vi "GeoData.vi"() -> ()   [LabVIEW 2017] (continued)
ND\tStark County\tH1\n58622\t38089\tBelfield\tND\tStark County\tH1\n58641\t38089\tLefor\tND\tStark County\tH1\n58602\t38089\tDickinson\tND\tStark County\tH1\n58652\t38089\tRichardton\tND\tStark County\tH1\n58630\t38089\tGladstone\tND\tStark County\tH1\n58274\t38091\tPortland\tND\tSteele County\tH1\n58035\t38091\tGalesburg\tND\tSteele County\tH1\n58056\t38091\tLuverne\tND\tSteele County\tH1\n58267\t38091\tNorthwood\tND\tSteele County\tH1\n58240\t38091\tHatton\tND\tSteele County\tH1\n58016\t38091\tClifford\tND\tSteele County\tH1\n58277\t38091\tSharon\tND\tSteele County\tH1\n58046\t38091\tHope\tND\tSteele County\tH1\n58230\t38091\tFinley\tND\tSteele County\tH1\n58425\t38091\tCooperstown\tND\tSteele County\tH1\n58401\t38093\tJamestown\tND\tStutsman County\tH1\n58492\t38093\tWimbledon\tND\tStutsman County\tH1\n58472\t38093\tMontpelier\tND\tStutsman County\tH1\n58420\t38093\tBuchanan\tND\tStutsman County\tH1\n58421\t38093\tCarrington\tND\tStutsman County\tH1\n58467\t38093\tMedina\tND\tStutsman County\tH1\n58466\t38093\tMarion\tND\tStutsman County\tH1\n58481\t38093\tSpiritwood\tND\tStutsman County\tH1\n58402\t38093\tJamestown\tND\tStutsman County\tH1\n58476\t38093\tPingree\tND\tStutsman County\tH1\n58483\t38093\tStreeter\tND\tStutsman County\tH1\n58497\t38093\tYpsilanti\tND\tStutsman County\tH1\n58426\t38093\tCourtenay\tND\tStutsman County\tH1\n58475\t38093\tPettibone\tND\tStutsman County\tH1\n58454\t38093\tJud\tND\tStutsman County\tH1\n58405\t38093\tJamestown\tND\tStutsman County\tH1\n58496\t38093\tWoodworth\tND\tStutsman County\tH1\n58424\t38093\tCleveland\tND\tStutsman County\tH1\n58455\t38093\tKensal\tND\tStutsman County\tH1\n58486\t38093\tSykeston\tND\tStutsman County\tH1\n58442\t38093\tGackle\tND\tStutsman County\tH1\n58367\t38095\tRolla\tND\tTowner County\tH1\n58324\t38095\tCando\tND\tTowner County\tH1\n58377\t38095\tStarkweather\tND\tTowner County\tH1\n58339\t38095\tHansboro\tND\tTowner County\tH1\n58352\t38095\tMunich\tND\tTowner County\tH1\n58331\t38095\tEgeland\tND\tTowner County\tH1\n58363\t38095\tPerth\tND\tTowner County\tH1\n58365\t38095\tRocklake\tND\tTowner County\tH1\n58325\t38095\tChurchs ferry\tND\tTowner County\tH1\n58317\t38095\tBisbee\tND\tTowner County\tH1\n58310\t38095\tAgate\tND\tTowner County\tH1\n58346\t38095\tLeeds\tND\tTowner County\tH1\n58372\t38095\tSarles\tND\tTowner County\tH1\n58323\t38095\tCalvin\tND\tTowner County\tH1\n58045\t38097\tHillsboro\tND\tTraill County\tH1\n58274\t38097\tPortland\tND\tTraill County\tH1\n58038\t38097\tGrandin\tND\tTraill County\tH1\n58218\t38097\tBuxton\tND\tTraill County\tH1\n58035\t38097\tGalesburg\tND\tTraill County\tH1\n58009\t38097\tBlanchard\tND\tTraill County\tH1\n58275\t38097\tReynolds\tND\tTraill County\tH1\n58223\t38097\tCummings\tND\tTraill County\tH1\n58240\t38097\tHatton\tND\tTraill County\tH1\n58016\t38097\tClifford\tND\tTraill County\tH1\n58048\t38097\tHunter\tND\tTraill County\tH1\n58257\t38097\tMayville\tND\tTraill County\tH1\n58219\t38097\tCaledonia\tND\tTraill County\tH1\n58259\t38099\tMichigan\tND\tWalsh County\tH1\n58261\t38099\tMinto\tND\tWalsh County\tH1\n58250\t38099\tLankin\tND\tWalsh County\tH1\n58330\t38099\tEdmore\tND\tWalsh County\tH1\n58321\t38099\tBrocket\tND\tWalsh County\tH1\n58227\t38099\tEdinburg\tND\tWalsh County\tH1\n58237\t38099\tGrafton\tND\tWalsh County\tH1\n58231\t38099\tFordville\tND\tWalsh County\tH1\n58224\t38099\tDahlen\tND\tWalsh County\tH1\n58345\t38099\tLawton\tND\tWalsh County\tH1\n58273\t38099\tPisek\tND\tWalsh County\tH1\n58270\t38099\tPark river\tND\tWalsh County\tH1\n58210\t38099\tAdams\tND\tWalsh County\tH1\n58243\t38099\tHoople\tND\tWalsh County\tH1\n58229\t38099\tFairdale\tND\tWalsh County\tH1\n58225\t38099\tDrayton\tND\tWalsh County\tH1\n58233\t38099\tForest river\tND\tWalsh County\tH1\n58779\t38101\tRyder\tND\tWard County\tH1\n58768\t38101\tNorwich\tND\tWard County\tH1\n58731\t38101\tDeering\tND\tWard County\tH1\n58759\t38101\tMax\tND\tWard County\tH1\n58740\t38101\tGlenburn\tND\tWard County\tH1\n58771\t38101\tPlaza\tND\tWard County\tH1\n58756\t38101\tMakoti\tND\tWard County\tH1\n58707\t38101\tMinot\tND\tWard County\tH1\n58704\t38101\tMinot afb\tND\tWard County\tH1\n58718\t38101\tBerthold\tND\tWard County\tH1\n58716\t38101\tBenedict\tND\tWard County\tH1\n58734\t38101\tDonnybrook\tND\tWard County\tH1\n58787\t38101\tTolley\tND\tWard County\tH1\n58721\t38101\tBowbells\tND\tWard County\tH1\n58781\t38101\tSawyer\tND\tWard County\tH1\n58725\t38101\tCarpio\tND\tWard County\tH1\n58733\t38101\tDes lacs\tND\tWard County\tH1\n58703\t38101\tMinot\tND\tWard County\tH1\n58722\t38101\tBurlington\tND\tWard County\tH1\n58790\t38101\tVelva\tND\tWard County\tH1\n58702\t38101\tMinot\tND\tWard County\tH1\n58735\t38101\tDouglas\tND\tWard County\tH1\n58705\t38101\tMinot afb\tND\tWard County\tH1\n58701\t38101\tMinot\tND\tWard County\tH1\n58746\t38101\tKenmare\tND\tWard County\tH1\n58785\t38101\tSurrey\tND\tWard County\tH1\n58374\t38103\tSheyenne\tND\tWells County\tH1\n58348\t38103\tMaddock\tND\tWells County\tH1\n58421\t38103\tCarrington\tND\tWells County\tH1\n58438\t38103\tFessenden\tND\tWells County\tH1\n58422\t38103\tCathay\tND\tWells County\tH1\n58418\t38103\tBowdon\tND\tWells County\tH1\n58356\t38103\tNew rockford\tND\tWells County\tH1\n58423\t38103\tChaseley\tND\tWells County\tH1\n58341\t38103\tHarvey\tND\tWells County\tH1\n58758\t38103\tMartin\tND\tWells County\tH1\n58486\t38103\tSykeston\tND\tWells County\tH1\n58451\t38103\tHurdsfield\tND\tWells County\tH1\n58801\t38105\tWilliston\tND\tWilliams County\tH1\n58849\t38105\tRay\tND\tWilliams County\tH1\n58845\t38105\tGrenora\tND\tWilliams County\tH1\n58843\t38105\tEpping\tND\tWilliams County\tH1\n58802\t38105\tWilliston\tND\tWilliams County\tH1\n58856\t38105\tZahl\tND\tWilliams County\tH1\n58755\t38105\tMcgregor\tND\tWilliams County\tH1\n58830\t38105\tAlamo\tND\tWilliams County\tH1\n58795\t38105\tWildrose\tND\tWilliams County\tH1\n58803\t38105\tWilliston\tND\tWilliams County\tH1\n58853\t38105\tTrenton\tND\tWilliams County\tH1\n58794\t38105\tWhite earth\tND\tWilliams County\tH1\n58852\t38105\tTioga\tND\tWilliams County\tH1\n45660\t39001\tPeebles\tOH\tAdams County\tH1\n45693\t39001\tWest union\tOH\tAdams County\tH1\n45144\t39001\tManchester\tOH\tAdams County\tH1\n45618\t39001\tCherry fork\tOH\tAdams County\tH1\n45616\t39001\tBlue creek\tOH\tAdams County\tH1\n45697\t39001\tWinchester\tOH\tAdams County\tH1\n45684\t39001\tStout\tOH\tAdams County\tH1\n45650\t39001\tLynx\tOH\tAdams County\tH1\n45101\t39001\tAberdeen\tOH\tAdams County\tH1\n45679\t39001\tSeaman\tOH\tAdams County\tH1\n45671\t39001\tRarden\tOH\tAdams County\tH1\n45105\t39001\tBentonville\tOH\tAdams County\tH1\n45657\t39001\tOtway\tOH\tAdams County\tH1\n45801\t39003\tLima\tOH\tAllen County\tH1\n45810\t39003\tAda\tOH\tAllen County\tH1\n45830\t39003\tColumbus grove\tOH\tAllen County\tH1\n45806\t39003\tLima\tOH\tAllen County\tH1\n45807\t39003\tLima\tOH\tAllen County\tH1\n45850\t39003\tHarrod\tOH\tAllen County\tH1\n45877\t39003\tPandora\tOH\tAllen County\tH1\n43310\t39003\tBelle center\tOH\tAllen County\tH1\n45802\t39003\tLima\tOH\tAllen County\tH1\n45854\t39003\tLafayette\tOH\tAllen County\tH1\n45895\t39003\tWapakoneta\tOH\tAllen County\tH1\n45896\t39003\tWaynesfield\tOH\tAllen County\tH1\n45833\t39003\tDelphos\tOH\tAllen County\tH1\n45805\t39003\tLima\tOH\tAllen County\tH1\n45881\t39003\tRawson\tOH\tAllen County\tH1\n45844\t39003\tFort jennings\tOH\tAllen County\tH1\n45820\t39003\tCairo\tOH\tAllen County\tH1\n45817\t39003\tBluffton\tOH\tAllen County\tH1\n45808\t39003\tBeaverdam\tOH\tAllen County\tH1\n45894\t39003\tVenedocia\tOH\tAllen County\tH1\n45887\t39003\tSpencerville\tOH\tAllen County\tH1\n45809\t39003\tGomer\tOH\tAllen County\tH1\n45804\t39003\tLima\tOH\tAllen County\tH1\n45812\t39003\tAlger\tOH\tAllen County\tH1\n44843\t39005\tLucas\tOH\tAshland County\tH1\n44864\t39005\tPerrysville\tOH\tAshland County\tH1\n44859\t39005\tNova\tOH\tAshland County\tH1\n44866\t39005\tPolk\tOH\tAshland County\tH1\n44287\t39005\tWest salem\tOH\tAshland County\tH1\n44691\t39005\tWooster\tOH\tAshland County\tH1\n44805\t39005\tAshland\tOH\tAshland County\tH1\n44837\t39005\tGreenwich\tOH\tAshland County\tH1\n44235\t39005\tHomerville\tOH\tAshland County\tH1\n44822\t39005\tButler\tOH\tAshland County\tH1\n44838\t39005\tHayesville\tOH\tAshland County\tH1\n44874\t39005\tSavannah\tOH\tAshland County\tH1\n44903\t39005\tMansfield\tOH\tAshland County\tH1\n44878\t39005\tShiloh\tOH\tAshland County\tH1\n44851\t39005\tNew london\tOH\tAshland County\tH1\n44842\t39005\tLoudonville\tOH\tAshland County\tH1\n44880\t39005\tSullivan\tOH\tAshland County\tH1\n44840\t39005\tJeromesville\tOH\tAshland County\tH1\n44848\t39005\tNankin\tOH\tAshland County\tH1\n44638\t39005\tLakeville\tOH\tAshland County\tH1\n44048\t39007\tKingsville\tOH\tAshtabula County\tH1\n44041\t39007\tGeneva\tOH\tAshtabula County\tH1\n44047\t39007\tJefferson\tOH\tAshtabula County\tH1\n44085\t39007\tRome\tOH\tAshtabula County\tH1\n44082\t39007\tPierpont\tOH\tAshtabula County\tH1\n44086\t39007\tThompson\tOH\tAshtabula County\tH1\n44046\t39007\tHuntsburg\tOH\tAshtabula County\tH1\n44084\t39007\tRock creek\tOH\tAshtabula County\tH1\n44032\t39007\tDorset\tOH\tAshtabula County\tH1\n44004\t39007\tAshtabula\tOH\tAshtabula County\tH1\n44003\t39007\tAndover\tOH\tAshtabula County\tH1\n44068\t39007\tNorth kingsville\tOH\tAshtabula County\tH1\n44062\t39007\tMiddlefield\tOH\tAshtabula County\tH1\n44428\t39007\tKinsman\tOH\tAshtabula County\tH1\n44076\t39007\tOrwell\tOH\tAshtabula County\tH1\n44010\t39007\tAustinburg\tOH\tAshtabula County\tH1\n44057\t39007\tMadison\tOH\tAshtabula County\tH1\n44093\t39007\tWilliamsfield\tOH\tAshtabula County\tH1\n44030\t39007\tConneaut\tOH\tAshtabula County\tH1\n44099\t39007\tWindsor\tOH\tAshtabula County\tH1\n44064\t39007\tMontville\tOH\tAshtabula County\tH1\n44088\t39007\tUnionville\tOH\tAshtabula County\tH1\n45701\t39009\tAthens\tOH\tAthens County\tH1\n45778\t39009\tStewart\tOH\tAthens County\tH1\n45780\t39009\tThe plains\tOH\tAthens County\tH1\n45723\t39009\tCoolville\tOH\tAthens County\tH1\n45766\t39009\tNew marshfield\tOH\tAthens County\tH1\n45782\t39009\tTrimble\tOH\tAthens County\tH1\n45776\t39009\tShade\tOH\tAthens County\tH1\n45711\t39009\tAmesville\tOH\tAthens County\tH1\n45732\t39009\tGlouster\tOH\tAthens County\tH1\n45764\t39009\tNelsonville\tOH\tAthens County\tH1\n45735\t39009\tGuysville\tOH\tAthens County\tH1\n45739\t39009\tHockingport\tOH\tAthens County\tH1\n43728\t39009\tChesterhill\tOH\tAthens County\tH1\n45710\t39009\tAlbany\tOH\tAthens County\tH1\n45742\t39009\tLittle hocking\tOH\tAthens County\tH1\n45761\t39009\tMillfield\tOH\tAthens County\tH1\n45716\t39009\tBuchtel\tOH\tAthens County\tH1\n45740\t39009\tJacksonville\tOH\tAthens County\tH1\n45719\t39009\tChauncey\tOH\tAthens County\tH1\n45801\t39011\tLima\tOH\tAuglaize County\tH1\n45865\t39011\tMinster\tOH\tAuglaize County\tH1\n43331\t39011\tLakeview\tOH\tAuglaize County\tH1\n45862\t39011\tMendon\tOH\tAuglaize County\tH1\n45806\t39011\tLima\tOH\tAuglaize County\tH1\n45850\t39011\tHarrod\tOH\tAuglaize County\tH1\n45888\t39011\tUniopolis\tOH\tAuglaize County\tH1\n45306\t39011\tBotkins\tOH\tAuglaize County\tH1\n45854\t39011\tLafayette\tOH\tAuglaize County\tH1\n45822\t39011\tCelina\tOH\tAuglaize County\tH1\n45895\t39011\tWapakoneta\tOH\tAuglaize County\tH1\n45896\t39011\tWaynesfield\tOH\tAuglaize County\tH1\n45871\t39011\tNew knoxville\tOH\tAuglaize County\tH1\n45869\t39011\tNew bremen\tOH\tAuglaize County\tH1\n45819\t39011\tBuckland\tOH\tAuglaize County\tH1\n45885\t39011\tSaint marys\tOH\tAuglaize County\tH1\n45887\t39011\tSpencerville\tOH\tAuglaize County\tH1\n45334\t39011\tJackson center\tOH\tAuglaize County\tH1\n45884\t39011\tSaint johns\tOH\tAuglaize County\tH1\n45845\t39011\tFort loramie\tOH\tAuglaize County\tH1\n45870\t39011\tNew hampshire\tOH\tAuglaize County\tH1\n43906\t39013\tBellaire\tOH\tBelmont County\tH1\n43917\t39013\tDillonvale\tOH\tBelmont County\tH1\n43977\t39013\tFlushing\tOH\tBelmont County\tH1\n43902\t39013\tAlledonia\tOH\tBelmont County\tH1\n43942\t39013\tPowhatan point\tOH\tBelmont County\tH1\n43719\t39013\tBethesda\tOH\tBelmont County\tH1\n43940\t39013\tNeffs\tOH\tBelmont County\tH1\n43943\t39013\tRayland\tOH\tBelmont County\tH1\n43935\t39013\tMartins ferry\tOH\tBelmont County\tH1\n43716\t39013\tBeallsville\tOH\tBelmont County\tH1\n43983\t39013\tPiedmont\tOH\tBelmont County\tH1\n43773\t39013\tQuaker city\tOH\tBelmont County\tH1\n43747\t39013\tJerusalem\tOH\tBelmont County\tH1\n43912\t39013\tBridgeport\tOH\tBelmont County\tH1\n43901\t39013\tAdena\tOH\tBelmont County\tH1\n43973\t39013\tFreeport\tOH\tBelmont County\tH1\n43933\t39013\tJacobsburg\tOH\tBelmont County\tH1\n43985\t39013\tHolloway\tOH\tBelmont County\tH1\n43927\t39013\tFairpoint\tOH\tBelmont County\tH1\n43916\t39013\tColerain\tOH\tBelmont County\tH1\n43905\t39013\tBarton\tOH\tBelmont County\tH1\n43972\t39013\tBannock\tOH\tBelmont County\tH1\n43934\t39013\tLansing\tOH\tBelmont County\tH1\n43971\t39013\tYorkville\tOH\tBelmont County\tH1\n43947\t39013\tShadyside\tOH\tBelmont County\tH1\n43718\t39013\tBelmont\tOH\tBelmont County\tH1\n43951\t39013\tLafferty\tOH\tBelmont County\tH1\n43937\t39013\tMaynard\tOH\tBelmont County\tH1\n43909\t39013\tBlaine\tOH\tBelmont County\tH1\n43950\t39013\tSaint clairsville\tOH\tBelmont County\tH1\n43713\t39013\tBarnesville\tOH\tBelmont County\tH1\n43967\t39013\tWarnock\tOH\tBelmont County\tH1\n43759\t39013\tMorristown\tOH\tBelmont County\tH1\n43928\t39013\tGlencoe\tOH\tBelmont County\tH1\n45119\t39015\tFeesburg\tOH\tBrown County\tH1\n45144\t39015\tManchester\tOH\tBrown County\tH1\n45167\t39015\tRipley\tOH\tBrown County\tH1\n45118\t39015\tFayetteville\tOH\tBrown County\tH1\n45142\t39015\tLynchburg\tOH\tBrown County\tH1\n45148\t39015\tMidland\tOH\tBrown County\tH1\n45121\t39015\tGeorgetown\tOH\tBrown County\tH1\n45697\t39015\tWinchester\tOH\tBrown County\tH1\n45154\t39015\tMount orab\tOH\tBrown County\tH1\n45107\t39015\tBlanchester\tOH\tBrown County\tH1\n45130\t39015\tHamersville\tOH\tBrown County\tH1\n45131\t39015\tHigginsport\tOH\tBrown County\tH1\n45171\t39015\tSardinia\tOH\tBrown County\tH1\n45106\t39015\tBethel\tOH\tBrown County\tH1\n45101\t39015\tAberdeen\tOH\tBrown County\tH1\n45115\t39015\tDecatur\tOH\tBrown County\tH1\n45176\t39015\tWilliamsburg\tOH\tBrown County\tH1\n45133\t39015\tHillsboro\tOH\tBrown County\tH1\n45120\t39015\tFelicity\tOH\tBrown County\tH1\n45168\t39015\tRussellville\tOH\tBrown County\tH1\n45005\t39017\tFranklin\tOH\tButler County\tH1\n45013\t39017\tHamilton\tOH\tButler County\tH1\n45014\t39017\tFairfield\tOH\tButler County\tH1\n45249\t39017\tCincinnati\tOH\tButler County\tH1\n45018\t39017\tFairfield\tOH\tButler County\tH1\n45003\t39017\tCollege corner\tOH\tButler County\tH1\n45069\t39017\tWest chester\tOH\tButler County\tH1\n45067\t39017\tTrenton\tOH\tButler County\tH1\n45071\t39017\tWest chester\tOH\tButler County\tH1\n45053\t39017\tOkeana\tOH\tButler County\tH1\n45030\t39017\tHarrison\tOH\tButler County\tH1\n45327\t39017\tGermantown\tOH\tButler County\tH1\n45063\t39017\tShandon\tOH\tButler County\tH1\n45004\t39017\tCollinsville\tOH\tButler County\tH1\n45064\t39017\tSomerville\tOH\tButler County\tH1\n45062\t39017\tSeven mile\tOH\tButler County\tH1\n45055\t39017\tOverpeck\tOH\tButler County\tH1\n45015\t39017\tHamilton\tOH\tButler County\tH1\n45042\t39017\tMiddletown\tOH\tButler County\tH1\n45044\t39017\tMiddletown\tOH\tButler County\tH1\n45050\t39017\tMonroe\tOH\tButler County\tH1\n45246\t39017\tCincinnati\tOH\tButler County\tH1\n45061\t39017\tRoss\tOH\tButler County\tH1\n45011\t39017\tHamilton\tOH\tButler County\tH1\n45056\t39017\tOxford\tOH\tButler County\tH1\n45241\t39017\tCincinnati\tOH\tButler County\tH1\n45012\t39017\tHamilton\tOH\tButler County\tH1\n44657\t39019\tMinerva\tOH\tCarroll County\tH1\n44695\t39019\tBowerston\tOH\tCarroll County\tH1\n44620\t39019\tDellroy\tOH\tCarroll County\tH1\n44644\t39019\tMalvern\tOH\tCarroll County\tH1\n44607\t39019\tAugusta\tOH\tCarroll County\tH1\n43988\t39019\tScio\tOH\tCarroll County\tH1\n44656\t39019\tMineral city\tOH\tCarroll County\tH1\n44643\t39019\tMagnolia\tOH\tCarroll County\tH1\n43908\t39019\tBergholz\tOH\tCarroll County\tH1\n44621\t39019\tDennison\tOH\tCarroll County\tH1\n44615\t39019\tCarrollton\tOH\tCarroll County\tH1\n43945\t39019\tSalineville\tOH\tCarroll County\tH1\n44651\t39019\tMechanicstown\tOH\tCarroll County\tH1\n44688\t39019\tWaynesburg\tOH\tCarroll County\tH1\n44625\t39019\tEast rochester\tOH\tCarroll County\tH1\n44639\t39019\tLeesville\tOH\tCarroll County\tH1\n43903\t39019\tAmsterdam\tOH\tCarroll County\tH1\n43986\t39019\tJewett\tOH\tCarroll County\tH1\n44730\t39019\tEast canton\tOH\tCarroll County\tH1\n44675\t39019\tSherrodsville\tOH\tCarroll County\tH1\n44427\t39019\tKensington\tOH\tCarroll County\tH1\n43047\t39021\tMingo\tOH\tChampaign County\tH1\n45502\t39021\tSpringfield\tOH\tChampaign County\tH1\n43070\t39021\tRosewood\tOH\tChampaign County\tH1\n43357\t39021\tWest liberty\tOH\tChampaign County\tH1\n45317\t39021\tConover\tOH\tChampaign County\tH1\n43060\t39021\tNorth lewisburg\tOH\tChampaign County\tH1\n43009\t39021\tCable\tOH\tChampaign County\tH1\n43045\t39021\tMilford center\tOH\tChampaign County\tH1\n43083\t39021\tWestville\tOH\tChampaign County\tH1\n45389\t39021\tChristiansburg\tOH\tChampaign County\tH1\n43078\t39021\tUrbana\tOH\tChampaign County\tH1\n43072\t39021\tSaint paris\tOH\tChampaign County\tH1\n43343\t39021\tQuincy\tOH\tChampaign County\tH1\n43318\t39021\tDe graff\tOH\tChampaign County\tH1\n45344\t39021\tNew carlisle\tOH\tChampaign County\tH1\n45365\t39021\tSidney\tOH\tChampaign County\tH1\n43044\t39021\tMechanicsburg\tOH\tChampaign County\tH1\n45312\t39021\tCasstown\tOH\tChampaign County\tH1\n43084\t39021\tWoodstock\tOH\tChampaign County\tH1\n45501\t39023\tSpringfield\tOH\tClark County\tH1\n45369\t39023\tSouth vienna\tOH\tClark County\tH1\n45387\t39023\tYellow springs\tOH\tClark County\tH1\n45502\t39023\tSpringfield\tOH\tClark County\tH1\n45319\t39023\tDonnelsville\tOH\tClark County\tH1\n43140\t39023\tLondon\tOH\tClark County\tH1\n45504\t39023\tSpringfield\tOH\tClark County\tH1\n43153\t39023\tSouth solon\tOH\tClark County\tH1\n45372\t39023\tTremont city\tOH\tClark County\tH1\n43078\t39023\tUrbana\tOH\tClark County\tH1\n45368\t39023\tSouth charleston\tOH\tClark County\tH1\n45349\t39023\tNorth hampton\tOH\tClark County\tH1\n45344\t39023\tNew carlisle\tOH\tClark County\tH1\n45314\t39023\tCedarville\tOH\tClark County\tH1\n45323\t39023\tEnon\tOH\tClark County\tH1\n45503\t39023\tSpringfield\tOH\tClark County\tH1\n45506\t39023\tSpringfield\tOH\tClark County\tH1\n43010\t39023\tCatawba\tOH\tClark County\tH1\n43044\t39023\tMechanicsburg\tOH\tClark County\tH1\n45324\t39023\tFairborn\tOH\tClark County\tH1\n45312\t39023\tCasstown\tOH\tClark County\tH1\n45341\t39023\tMedway\tOH\tClark County\tH1\n45505\t39023\tSpringfield\tOH\tClark County\tH1\n45153\t39025\tMoscow\tOH\tClermont County\tH1\n45255\t39025\tCincinnati\tOH\tClermont County\tH1\n45147\t39025\tMiamiville\tOH\tClermont County\tH1\n45103\t39025\tBatavia\tOH\tClermont County\tH1\n45150\t39025\tMilford\tOH\tClermont County\tH1\n45118\t39025\tFayetteville\tOH\tClermont County\tH1\n45162\t39025\tPleasant plain\tOH\tClermont County\tH1\n45121\t39025\tGeorgetown\tOH\tClermont County\tH1\n45156\t39025\tNeville\tOH\tClermont County\tH1\n45112\t39025\tChilo\tOH\tClermont County\tH1\n45107\t39025\tBlanchester\tOH\tClermont County\tH1\n45130\t39025\tHamersville\tOH\tClermont County\tH1\n45102\t39025\tAmelia\tOH\tClermont County\tH1\n45122\t39025\tGoshen\tOH\tClermont County\tH1\n45157\t39025\tNew richmond\tOH\tClermont County\tH1\n45106\t39025\tBethel\tOH\tClermont County\tH1\n45244\t39025\tCincinnati\tOH\tClermont County\tH1\n45176\t39025\tWilliamsburg\tOH\tClermont County\tH1\n45120\t39025\tFelicity\tOH\tClermont County\tH1\n45245\t39025\tCincinnati\tOH\tClermont County\tH1\n45140\t39025\tLoveland\tOH\tClermont County\tH1\n45160\t39025\tOwensville\tOH\tClermont County\tH1\n45158\t39025\tNewtonsville\tOH\tClermont County\tH1\n45177\t39027\tWilmington\tOH\tClinton County\tH1\n45164\t39027\tPort william\tOH\tClinton County\tH1\n45142\t39027\tLynchburg\tOH\tClinton County\tH1\n45148\t39027\tMidland\tOH\tClinton County\tH1\n45159\t39027\tNew vienna\tOH\tClinton County\tH1\n45169\t39027\tSabina\tOH\tClinton County\tH1\n45385\t39027\tXenia\tOH\tClinton County\tH1\n45146\t39027\tMartinsville\tOH\tClinton County\tH1\n45107\t39027\tBlanchester\tOH\tClinton County\tH1\n45068\t39027\tWaynesville\tOH\tClinton County\tH1\n45113\t39027\tClarksville\tOH\tClinton County\tH1\n45135\t39027\tLeesburg\tOH\tClinton County\tH1\n45335\t39027\tJamestown\tOH\tClinton County\tH1\n45114\t39027\tCuba\tOH\tClinton County\tH1\n43160\t39027\tWashington court house\tOH\tClinton County\tH1\n45166\t39027\tReesville\tOH\tClinton County\tH1\n44657\t39029\tMinerva\tOH\tColumbiana County\tH1\n44455\t39029\tRogers\tOH\tColumbiana County\tH1\n44493\t39029\tWinona\tOH\tColumbiana County\tH1\n44454\t39029\tPetersburg\tOH\tColumbiana County\tH1\n44415\t39029\tElkton\tOH\tColumbiana County\tH1\n44460\t39029\tSalem\tOH\tColumbiana County\tH1\n44408\t39029\tColumbiana\tOH\tColumbiana County\tH1\n44413\t39029\tEast palestine\tOH\tColumbiana County\tH1\n43930\t39029\tHammondsville\tOH\tColumbiana County\tH1\n43962\t39029\tSummitville\tOH\tColumbiana County\tH1\n43945\t39029\tSalineville\tOH\tColumbiana County\tH1\n44634\t39029\tHomeworth\tOH\tColumbiana County\tH1\n44625\t39029\tEast rochester\tOH\tColumbiana County\tH1\n43932\t39029\tIrondale\tOH\tColumbiana County\tH1\n44431\t39029\tLeetonia\tOH\tColumbiana County\tH1\n44445\t39029\tNew waterford\tOH\tColumbiana County\tH1\n44490\t39029\tWashingtonville\tOH\tColumbiana County\tH1\n44443\t39029\tNew springfield\tOH\tColumbiana County\tH1\n43968\t39029\tWellsville\tOH\tColumbiana County\tH1\n44601\t39029\tAlliance\tOH\tColumbiana County\tH1\n44427\t39029\tKensington\tOH\tColumbiana County\tH1\n43920\t39029\tEast liverpool\tOH\tColumbiana County\tH1\n44432\t39029\tLisbon\tOH\tColumbiana County\tH1\n44423\t39029\tHanoverton\tOH\tColumbiana County\tH1\n44441\t39029\tNegley\tOH\tColumbiana County\tH1\n44492\t39029\tWest point\tOH\tColumbiana County\tH1\n44609\t39029\tBeloit\tOH\tColumbiana County\tH1\n44665\t39029\tNorth georgetown\tOH\tColumbiana County\tH1\n43845\t39031\tWest lafayette\tOH\tCoshocton County\tH1\n43828\t39031\tKeene\tOH\tCoshocton County\tH1\n43824\t39031\tFresno\tOH\tCoshocton County\tH1\n43821\t39031\tDresden\tOH\tCoshocton County\tH1\n43749\t39031\tKimbolton\tOH\tCoshocton County\tH1\n44637\t39031\tKillbuck\tOH\tCoshocton County\tH1\n43811\t39031\tConesville\tOH\tCoshocton County\tH1\n43803\t39031\tBakersville\tOH\tCoshocton County\tH1\n44654\t39031\tMillersburg\tOH\tCoshocton County\tH1\n43804\t39031\tBaltic\tOH\tCoshocton County\tH1\n43812\t39031\tCoshocton\tOH\tCoshocton County\tH1\n43832\t39031\tNewcomerstown\tOH\tCoshocton County\tH1\n43844\t39031\tWarsaw\tOH\tCoshocton County\tH1\n43822\t39031\tFrazeysburg\tOH\tCoshocton County\tH1\n43006\t39031\tBrinkhaven\tOH\tCoshocton County\tH1\n43805\t39031\tBlissfield\tOH\tCoshocton County\tH1\n43840\t39031\tStone creek\tOH\tCoshocton County\tH1\n43843\t39031\tWalhonding\tOH\tCoshocton County\tH1\n43836\t39031\tPlainfield\tOH\tCoshocton County\tH1\n44827\t39033\tCrestline\tOH\tCrawford County\tH1\n44887\t39033\tTiro\tOH\tCrawford County\tH1\n44849\t39033\tNevada\tOH\tCrawford County\tH1\n44875\t39033\tShelby\tOH\tCrawford County\tH1\n44860\t39033\tOceola\tOH\tCrawford County\tH1\n43314\t39033\tCaledonia\tOH\tCrawford County\tH1\n44818\t39033\tBloomville\tOH\tCrawford County\tH1\n43302\t39033\tMarion\tOH\tCrawford County\tH1\n44881\t39033\tSulphur springs\tOH\tCrawford County\tH1\n44865\t39033\tPlymouth\tOH\tCrawford County\tH1\n44825\t39033\tChatfield\tOH\tCrawford County\tH1\n44833\t39033\tGalion\tOH\tCrawford County\tH1\n44854\t39033\tNew washington\tOH\tCrawford County\tH1\n44882\t39033\tSycamore\tOH\tCrawford County\tH1\n44856\t39033\tNorth robinson\tOH\tCrawford County\tH1\n44820\t39033\tBucyrus\tOH\tCrawford County\tH1\n44026\t39035\tChesterland\tOH\tCuyahoga County\tH1\n44130\t39035\tCleveland\tOH\tCuyahoga County\tH1\n44111\t39035\tCleveland\tOH\tCuyahoga County\tH1\n44113\t39035\tCleveland\tOH\tCuyahoga County\tH1\n44144\t39035\tCleveland\tOH\tCuyahoga County\tH1\n44102\t39035\tCleveland\tOH\tCuyahoga County\tH1\n44040\t39035\tGates mills\tOH\tCuyahoga County\tH1\n44017\t39035\tBerea\tOH\tCuyahoga County\tH1\n44124\t39035\tCleveland\tOH\tCuyahoga County\tH1\n44109\t39035\tCleveland\tOH\tCuyahoga County\tH1\n44127\t39035\tCleveland\tOH\tCuyahoga County\tH1\n44112\t39035\tCleveland\tOH\tCuyahoga County\tH1\n44136\t39035\tStrongsville\tOH\tCuyahoga County\tH1\n44138\t39035\tOlmsted falls\tOH\tCuyahoga County\tH1\n44143\t39035\tCleveland\tOH\tCuyahoga County\tH1\n44105\t39035\tCleveland\tOH\tCuyahoga County\tH1\n44023\t39035\tChagrin falls\tOH\tCuyahoga County\tH1\n44110\t39035\tCleveland\tOH\tCuyahoga County\tH1\n44117\t39035\tEuclid\tOH\tCuyahoga County\tH1\n44134\t39035\tCleveland\tOH\tCuyahoga County\tH1\n44233\t39035\tHinckley\tOH\tCuyahoga County\tH1\n44142\t39035\tBrookpark\tOH\tCuyahoga County\tH1\n44070\t39035\tNorth olmsted\tOH\tCuyahoga County\tH1\n44092\t39035\tWickliffe\tOH\tCuyahoga County\tH1\n44125\t39035\tCleveland\tOH\tCuyahoga County\tH1\n44116\t39035\tRocky river\tOH\tCuyahoga County\tH1\n44114\t39035\tCleveland\tOH\tCuyahoga County\tH1\n44147\t39035\tBroadview heights\tOH\tCuyahoga County\tH1\n44199\t39035\tCleveland\tOH\tCuyahoga County\tH1\n44123\t39035\tEuclid\tOH\tCuyahoga County\tH1\n44129\t39035\tCleveland\tOH\tCuyahoga County\tH1\n44131\t39035\tIndependence\tOH\tCuyahoga County\tH1\n44120\t39035\tCleveland\tOH\tCuyahoga County\tH1\n44128\t39035\tCleveland\tOH\tCuyahoga County\tH1\n44137\t39035\tMaple heights\tOH\tCuyahoga County\tH1\n44133\t39035\tNorth royalton\tOH\tCuyahoga County\tH1\n44140\t39035\tBay village\tOH\tCuyahoga County\tH1\n44141\t39035\tBrecksville\tOH\tCuyahoga County\tH1\n44104\t39035\tCleveland\tOH\tCuyahoga County\tH1\n44119\t39035\tCleveland\tOH\tCuyahoga County\tH1\n44122\t39035\tBeachwood\tOH\tCuyahoga County\tH1\n44135\t39035\tCleveland\tOH\tCuyahoga County\tH1\n44139\t39035\tSolon\tOH\tCuyahoga County\tH1\n44115\t39035\tCleveland\tOH\tCuyahoga County\tH1\n44106\t39035\tCleveland\tOH\tCuyahoga County\tH1\n44103\t39035\tCleveland\tOH\tCuyahoga County\tH1\n44022\t39035\tChagrin falls\tOH\tCuyahoga County\tH1\n44132\t39035\tEuclid\tOH\tCuyahoga County\tH1\n44149\t39035\tStrongsville\tOH\tCuyahoga County\tH1\n44145\t39035\tWestlake\tOH\tCuyahoga County\tH1\n44181\t39035\tCleveland\tOH\tCuyahoga County\tH1\n44126\t39035\tCleveland\tOH\tCuyahoga County\tH1\n44121\t39035\tCleveland\tOH\tCuyahoga County\tH1\n44118\t39035\tCleveland\tOH\tCuyahoga County\tH1\n44108\t39035\tCleveland\tOH\tCuyahoga County\tH1\n44146\t39035\tBedford\tOH\tCuyahoga County\tH1\n44107\t39035\tLakewood\tOH\tCuyahoga County\tH1\n44101\t39035\tCleveland\tOH\tCuyahoga County\tH1\n44195\t39035\tCleveland\tOH\tCuyahoga County\tH1\n45358\t39037\tPitsburg\tOH\tDarke County\tH1\n45383\t39037\tWest milton\tOH\tDarke County\tH1\n45304\t39037\tArcanum\tOH\tDarke County\tH1\n45382\t39037\tWest manchester\tOH\tDarke County\tH1\n45337\t39037\tLaura\tOH\tDarke County\tH1\n45883\t39037\tSaint henry\tOH\tDarke County\tH1\n45346\t39037\tNew madison\tOH\tDarke County\tH1\n45309\t39037\tBrookville\tOH\tDarke County\tH1\n45362\t39037\tRossburg\tOH\tDarke County\tH1\n45351\t39037\tOsgood\tOH\tDarke County\tH1\n45331\t39037\tGreenville\tOH\tDarke County\tH1\n45318\t39037\tCovington\tOH\tDarke County\tH1\n45388\t39037\tYorkshire\tOH\tDarke County\tH1\n45390\t39037\tUnion city\tOH\tDarke County\tH1\n45347\t39037\tNew paris\tOH\tDarke County\tH1\n45350\t39037\tNorth star\tOH\tDarke County\tH1\n45308\t39037\tBradford\tOH\tDarke County\tH1\n45303\t39037\tAnsonia\tOH\tDarke County\tH1\n45352\t39037\tPalestine\tOH\tDarke County\tH1\n45846\t39037\tFort recovery\tOH\tDarke County\tH1\n45332\t39037\tHollansburg\tOH\tDarke County\tH1\n45380\t39037\tVersailles\tOH\tDarke County\tH1\n45348\t39037\tNew weston\tOH\tDarke County\tH1\n45328\t39037\tGettysburg\tOH\tDarke County\tH1\n45845\t39037\tFort loramie\tOH\tDarke County\tH1\n43506\t39039\tBryan\tOH\tDefiance County\tH1\n43527\t39039\tHolgate\tOH\tDefiance County\tH1\n43530\t39039\tJewell\tOH\tDefiance County\tH1\n43536\t39039\tMark center\tOH\tDefiance County\tH1\n45813\t39039\tAntwerp\tOH\tDefiance County\tH1\n45831\t39039\tContinental\tOH\tDefiance County\tH1\n43549\t39039\tNey\tOH\tDefiance County\tH1\n43520\t39039\tFarmer\tOH\tDefiance County\tH1\n43548\t39039\tNew bavaria\tOH\tDefiance County\tH1\n45821\t39039\tCecil\tOH\tDefiance County\tH1\n43517\t39039\tEdgerton\tOH\tDefiance County\tH1\n43512\t39039\tDefiance\tOH\tDefiance County\tH1\n43526\t39039\tHicksville\tOH\tDefiance County\tH1\n43545\t39039\tNapoleon\tOH\tDefiance County\tH1\n43556\t39039\tSherwood\tOH\tDefiance County\tH1\n43519\t39039\tEvansport\tOH\tDefiance County\tH1\n43035\t39041\tLewis center\tOH\tDelaware County\tH1\n43064\t39041\tPlain city\tOH\tDelaware County\tH1\n43061\t39041\tOstrander\tOH\tDelaware County\tH1\n43334\t39041\tMarengo\tOH\tDelaware County\tH1\n43240\t39041\tColumbus\tOH\tDelaware County\tH1\n43066\t39041\tRadnor\tOH\tDelaware County\tH1\n43081\t39041\tWesterville\tOH\tDelaware County\tH1\n43065\t39041\tPowell\tOH\tDelaware County\tH1\n43031\t39041\tJohnstown\tOH\tDelaware County\tH1\n43344\t39041\tRichwood\tOH\tDelaware County\tH1\n43235\t39041\tColumbus\tOH\tDelaware County\tH1\n43015\t39041\tDelaware\tOH\tDelaware County\tH1\n43021\t39041\tGalena\tOH\tDelaware County\tH1\n43082\t39041\tWesterville\tOH\tDelaware County\tH1\n43054\t39041\tNew albany\tOH\tDelaware County\tH1\n43013\t39041\tCroton\tOH\tDelaware County\tH1\n43342\t39041\tProspect\tOH\tDelaware County\tH1\n43040\t39041\tMarysville\tOH\tDelaware County\tH1\n43074\t39041\tSunbury\tOH\tDelaware County\tH1\n43017\t39041\tDublin\tOH\tDelaware County\tH1\n43086\t39041\tWesterville\tOH\tDelaware County\tH1\n43003\t39041\tAshley\tOH\tDelaware County\tH1\n43016\t39041\tDublin\tOH\tDelaware County\tH1\n43011\t39041\tCenterburg\tOH\tDelaware County\tH1\n43356\t39041\tWaldo\tOH\tDelaware County\tH1\n44824\t39043\tCastalia\tOH\tErie County\tH1\n44847\t39043\tMonroeville\tOH\tErie County\tH1\n44889\t39043\tWakeman\tOH\tErie County\tH1\n44870\t39043\tSandusky\tOH\tErie County\tH1\n44839\t39043\tHuron\tOH\tErie County\tH1\n44814\t39043\tBerlin heights\tOH\tErie County\tH1\n43438\t39043\tKelleys island\tOH\tErie County\tH1\n44826\t39043\tCollins\tOH\tErie County\tH1\n43464\t39043\tVickery\tOH\tErie County\tH1\n44816\t39043\tBirmingham\tOH\tErie County\tH1\n44811\t39043\tBellevue\tOH\tErie County\tH1\n44871\t39043\tSandusky\tOH\tErie County\tH1\n44846\t39043\tMilan\tOH\tErie County\tH1\n44089\t39043\tVermilion\tOH\tErie County\tH1\n44857\t39043\tNorwalk\tOH\tErie County\tH1\n43076\t39045\tThornville\tOH\tFairfield County\tH1\n43148\t39045\tPleasantville\tOH\tFairfield County\tH1\n43155\t39045\tSugar grove\tOH\tFairfield County\tH1\n43107\t39045\tBremen\tOH\tFairfield County\tH1\n43105\t39045\tBaltimore\tOH\tFairfield County\tH1\n43112\t39045\tCarroll\tOH\tFairfield County\tH1\n43147\t39045\tPickerington\tOH\tFairfield County\tH1\n43110\t39045\tCanal winchester\tOH\tFairfield County\tH1\n43046\t39045\tMillersport\tOH\tFairfield County\tH1\n43102\t39045\tAmanda\tOH\tFairfield County\tH1\n43154\t39045\tStoutsville\tOH\tFairfield County\tH1\n43068\t39045\tReynoldsburg\tOH\tFairfield County\tH1\n43130\t39045\tLancaster\tOH\tFairfield County\tH1\n43136\t39045\tLithopolis\tOH\tFairfield County\tH1\n43103\t39045\tAshville\tOH\tFairfield County\tH1\n43113\t39045\tCircleville\tOH\tFairfield County\tH1\n43062\t39045\tPataskala\tOH\tFairfield County\tH1\n43157\t39045\tThurston\tOH\tFairfield County\tH1\n43150\t39045\tRushville\tOH\tFairfield County\tH1\n43145\t39047\tNew holland\tOH\tFayette County\tH1\n45169\t39047\tSabina\tOH\tFayette County\tH1\n43106\t39047\tBloomingburg\tOH\tFayette County\tH1\n43143\t39047\tMount sterling\tOH\tFayette County\tH1\n43153\t39047\tSouth solon\tOH\tFayette County\tH1\n43128\t39047\tJeffersonville\tOH\tFayette County\tH1\n45123\t39047\tGreenfield\tOH\tFayette County\tH1\n45135\t39047\tLeesburg\tOH\tFayette County\tH1\n45335\t39047\tJamestown\tOH\tFayette County\tH1\n43142\t39047\tMilledgeville\tOH\tFayette County\tH1\n43160\t39047\tWashington court house\tOH\tFayette County\tH1\n43064\t39049\tPlain city\tOH\tFranklin County\tH1\n43026\t39049\tHilliard\tOH\tFranklin County\tH1\n43220\t39049\tColumbus\tOH\tFranklin County\tH1\n43230\t39049\tColumbus\tOH\tFranklin County\tH1\n43209\t39049\tColumbus\tOH\tFranklin County\tH1\n43137\t39049\tLockbourne\tOH\tFranklin County\tH1\n43109\t39049\tBrice\tOH\tFranklin County\tH1\n43218\t39049\tColumbus\tOH\tFranklin County\tH1\n43081\t39049\tWesterville\tOH\tFranklin County\tH1\n43085\t39049\tColumbus\tOH\tFranklin County\tH1\n43065\t39049\tPowell\tOH\tFranklin County\tH1\n43223\t39049\tColumbus\tOH\tFranklin County\tH1\n43235\t39049\tColumbus\tOH\tFranklin County\tH1\n43004\t39049\tBlacklick\tOH\tFranklin County\tH1\n43126\t39049\tHarrisburg\tOH\tFranklin County\tH1\n43226\t39049\tColumbus\tOH\tFranklin County\tH1\n43287\t39049\tColumbus\tOH\tFranklin County\tH1\n43123\t39049\tGrove city\tOH\tFranklin County\tH1\n43147\t39049\tPickerington\tOH\tFranklin County\tH1\n43228\t39049\tColumbus\tOH\tFranklin County\tH1\n43203\t39049\tColumbus\tOH\tFranklin County\tH1\n43206\t39049\tColumbus\tOH\tFranklin County\tH1\n43202\t39049\tColumbus\tOH\tFranklin County\tH1\n43212\t39049\tColumbus\tOH\tFranklin County\tH1\n43195\t39049\tGroveport\tOH\tFranklin County\tH1\n43082\t39049\tWesterville\tOH\tFranklin County\tH1\n43110\t39049\tCanal winchester\tOH\tFranklin County\tH1\n43140\t39049\tLondon\tOH\tFranklin County\tH1\n43054\t39049\tNew albany\tOH\tFranklin County\tH1\n43216\t39049\tColumbus\tOH\tFranklin County\tH1\n43224\t39049\tColumbus\tOH\tFranklin County\tH1\n43201\t39049\tColumbus\tOH\tFranklin County\tH1\n43211\t39049\tColumbus\tOH\tFranklin County\tH1\n43232\t39049\tColumbus\tOH\tFranklin County\tH1\n43291\t39049\tColumbus\tOH\tFranklin County\tH1\n43068\t39049\tReynoldsburg\tOH\tFranklin County\tH1\n43119\t39049\tGalloway\tOH\tFranklin County\tH1\n43214\t39049\tColumbus\tOH\tFranklin County\tH1\n43205\t39049\tColumbus\tOH\tFranklin County\tH1\n43213\t39049\tColumbus\tOH\tFranklin County\tH1\n43210\t39049\tColumbus\tOH\tFranklin County\tH1\n43217\t39049\tColumbus\tOH\tFranklin County\tH1\n43215\t39049\tColumbus\tOH\tFranklin County\tH1\n43207\t39049\tColumbus\tOH\tFranklin County\tH1\n43231\t39049\tColumbus\tOH\tFranklin County\tH1\n43236\t39049\tColumbus\tOH\tFranklin County\tH1\n43062\t39049\tPataskala\tOH\tFranklin County\tH1\n43221\t39049\tColumbus\tOH\tFranklin County\tH1\n43229\t39049\tColumbus\tOH\tFranklin County\tH1\n43204\t39049\tColumbus\tOH\tFranklin County\tH1\n43017\t39049\tDublin\tOH\tFranklin County\tH1\n43086\t39049\tWesterville\tOH\tFranklin County\tH1\n43234\t39049\tColumbus\tOH\tFranklin County\tH1\n43002\t39049\tAmlin\tOH\tFranklin County\tH1\n43251\t39049\tColumbus\tOH\tFranklin County\tH1\n43146\t39049\tOrient\tOH\tFranklin County\tH1\n43125\t39049\tGroveport\tOH\tFranklin County\tH1\n43219\t39049\tColumbus\tOH\tFranklin County\tH1\n43227\t39049\tColumbus\tOH\tFranklin County\tH1\n43222\t39049\tColumbus\tOH\tFranklin County\tH1\n43016\t39049\tDublin\tOH\tFranklin County\tH1\n43194\t39049\tLockbourne\tOH\tFranklin County\tH1\n43069\t39049\tReynoldsburg\tOH\tFranklin County\tH1\n43533\t39051\tLyons\tOH\tFulton County\tH1\n43532\t39051\tLiberty center\tOH\tFulton County\tH1\n43504\t39051\tBerkey\tOH\tFulton County\tH1\n43570\t39051\tWest unity\tOH\tFulton County\tH1\n43521\t39051\tFayette\tOH\tFulton County\tH1\n43558\t39051\tSwanton\tOH\tFulton County\tH1\n43553\t39051\tPettisville\tOH\tFulton County\tH1\n43515\t39051\tDelta\tOH\tFulton County\tH1\n43567\t39051\tWauseon\tOH\tFulton County\tH1\n43502\t39051\tArchbold\tOH\tFulton County\tH1\n43557\t39051\tStryker\tOH\tFulton County\tH1\n43540\t39051\tMetamora\tOH\tFulton County\tH1\n43545\t39051\tNapoleon\tOH\tFulton County\tH1\n45623\t39053\tCrown city\tOH\tGallia County\tH1\n45658\t39053\tPatriot\tOH\tGallia County\tH1\n45688\t39053\tWaterloo\tOH\tGallia County\tH1\n45760\t39053\tMiddleport\tOH\tGallia County\tH1\n45614\t39053\tBidwell\tOH\tGallia County\tH1\n45674\t39053\tRio grande\tOH\tGallia County\tH1\n45686\t39053\tVinton\tOH\tGallia County\tH1\n45656\t39053\tOak hill\tOH\tGallia County\tH1\n45643\t39053\tKerr\tOH\tGallia County\tH1\n45631\t39053\tGallipolis\tOH\tGallia County\tH1\n45685\t39053\tThurman\tOH\tGallia County\tH1\n45620\t39053\tCheshire\tOH\tGallia County\tH1\n45678\t39053\tScottown\tOH\tGallia County\tH1\n44026\t39055\tChesterland\tOH\tGeauga County\tH1\n44040\t39055\tGates mills\tOH\tGeauga County\tH1\n44086\t39055\tThompson\tOH\tGeauga County\tH1\n44021\t39055\tBurton\tOH\tGeauga County\tH1\n44024\t39055\tChardon\tOH\tGeauga County\tH1\n44023\t39055\tChagrin falls\tOH\tGeauga County\tH1\n44060\t39055\tMentor\tOH\tGeauga County\tH1\n44094\t39055\tWilloughby\tOH\tGeauga County\tH1\n44046\t39055\tHuntsburg\tOH\tGeauga County\tH1\n44202\t39055\tAurora\tOH\tGeauga County\tH1\n44491\t39055\tWest farmington\tOH\tGeauga County\tH1\n44062\t39055\tMiddlefield\tOH\tGeauga County\tH1\n44080\t39055\tParkman\tOH\tGeauga County\tH1\n44022\t39055\tChagrin falls\tOH\tGeauga County\tH1\n44231\t39055\tGarrettsville\tOH\tGeauga County\tH1\n44057\t39055\tMadison\tOH\tGeauga County\tH1\n44065\t39055\tNewbury\tOH\tGeauga County\tH1\n44234\t39055\tHiram\tOH\tGeauga County\tH1\n44033\t39055\tEast claridon\tOH\tGeauga County\tH1\n44077\t39055\tPainesville\tOH\tGeauga County\tH1\n44072\t39055\tNovelty\tOH\tGeauga County\tH1\n44099\t39055\tWindsor\tOH\tGeauga County\tH1\n44064\t39055\tMontville\tOH\tGeauga County\tH1\n44073\t39055\tNovelty\tOH\tGeauga County\tH1\n45440\t39057\tDayton\tOH\tGreene County\tH1\n45430\t39057\tDayton\tOH\tGreene County\tH1\n45316\t39057\tClifton\tOH\tGreene County\tH1\n45387\t39057\tYellow springs\tOH\tGreene County\tH1\n45307\t39057\tBowersville\tOH\tGreene County\tH1\n45435\t39057\tDayton\tOH\tGreene County\tH1\n45169\t39057\tSabina\tOH\tGreene County\tH1\n45385\t39057\tXenia\tOH\tGreene County\tH1\n45433\t39057\tDayton\tOH\tGreene County\tH1\n45434\t39057\tDayton\tOH\tGreene County\tH1\n45384\t39057\tWilberforce\tOH\tGreene County\tH1\n45481\t39057\tDayton\tOH\tGreene County\tH1\n45305\t39057\tBellbrook\tOH\tGreene County\tH1\n43153\t39057\tSouth solon\tOH\tGreene County\tH1\n43128\t39057\tJeffersonville\tOH\tGreene County\tH1\n45424\t39057\tDayton\tOH\tGreene County\tH1\n45431\t39057\tDayton\tOH\tGreene County\tH1\n45368\t39057\tSouth charleston\tOH\tGreene County\tH1\n45068\t39057\tWaynesville\tOH\tGreene County\tH1\n45335\t39057\tJamestown\tOH\tGreene County\tH1\n45370\t39057\tSpring valley\tOH\tGreene County\tH1\n45314\t39057\tCedarville\tOH\tGreene County\tH1\n45458\t39057\tDayton\tOH\tGreene County\tH1\n45324\t39057\tFairborn\tOH\tGreene County\tH1\n45432\t39057\tDayton\tOH\tGreene County\tH1\n45459\t39057\tDayton\tOH\tGreene County\tH1\n45301\t39057\tAlpha\tOH\tGreene County\tH1\n43772\t39059\tPleasant city\tOH\tGuernsey County\tH1\n43837\t39059\tPort washington\tOH\tGuernsey County\tH1\n44699\t39059\tTippecanoe\tOH\tGuernsey County\tH1\n43750\t39059\tKipling\tOH\tGuernsey County\tH1\n43749\t39059\tKimbolton\tOH\tGuernsey County\tH1\n43762\t39059\tNew concord\tOH\tGuernsey County\tH1\n43733\t39059\tDerwent\tOH\tGuernsey County\tH1\n43724\t39059\tCaldwell\tOH\tGuernsey County\tH1\n43983\t39059\tPiedmont\tOH\tGuernsey County\tH1\n43773\t39059\tQuaker city\tOH\tGuernsey County\tH1\n43973\t39059\tFreeport\tOH\tGuernsey County\tH1\n43723\t39059\tByesville\tOH\tGuernsey County\tH1\n43755\t39059\tLore city\tOH\tGuernsey County\tH1\n43832\t39059\tNewcomerstown\tOH\tGuernsey County\tH1\n43725\t39059\tCambridge\tOH\tGuernsey County\tH1\n43780\t39059\tSenecaville\tOH\tGuernsey 
